vi "8-Axis RS Coordinate Move (bad).vi"() -> ()   [LabVIEW 2013]
uses:
  Typedef/Typedef_Motor_Message.ctl
  EMC API/EMC_Typedef_Motor_Parameters.ctl
  Functional_Global/Typedef_Message_Queue_Action.ctl
  Globals/Global Stop.vi
  <vilib>/Motion/Express/_s/nimc.ex.power.power.axis.vi
  <vilib>/Motion/Express/_s/nimc.ex.resetPosition.resetPosition.axis.vi
  <vilib>/Motion/Express/_s/nimc.ex.straightLineMove.startStraightLineMove.coordinate.modeRelative.0.vi
  Globals/Default Motor Parameters.vi
  <vilib>/Motion/Express/_s/nimc.ex.straightLineMove.startStraightLineMove.axis.modeRelative.0.vi
  <vilib>/Motion/Express/_s/nimc.ex.stopMove.stop.coordinate.modeDecelerate.vi
  <vilib>/Motion/Express/_s/nimc.ex.stopMove.stop.axis.modeDecelerate.vi
  <vilib>/Motion/Express/_s/nimc.ex.read.readTrajectoryData.axis.vi
  <vilib>/Motion/BlockNode/FB.NIMotion.xnode
  Functional_Global/Typedef_FPGA_Interface_Action.ctl
  support/Message Queue/Message Queue.lvlib
  Typedef/Typedef_Coordinate_Move_Message.ctl
panel:
  in  "velocity 3":dbl=1000.0
  in  "position":dbl=1000.0
  in  "velocity 2":dbl=1000.0
  in  "position[]":dbl[](array[numeric])
  in  "Stop all motors 2":bool
  out "error out 2":errorcluster
  in  "velocity":dbl
  in  "# whole revs":dbl=3.0 format="%#_13g"
  in  "Auto Cycle Time (s)":dbl=10.0 format="%#_13g"
  in  "Auto":bool=TRUE
  in  "Mode":enum16{"Seq 1", "Seq 2", "Seq 3"}(ring)
  in  "cts per rev":dbl=1600.0 format="%#_13g"
  in  "Stop all motors":bool
  in  "Max delay (ms)":u32=1000
  in  "Motion Parameters (Min)":T1={"position"=-10000.0, "velocity"=-10000.0, "acceleration"=50000.0, "deceleration"=50000.0, "accel. jerk"=800000.0, "decel. jerk"=800000.0}
  in  "Motion Parameters (Max)":T1={"position"=10000.0, "velocity"=10000.0, "acceleration"=100000.0, "deceleration"=100000.0, "accel. jerk"=1000000.0, "decel. jerk"=1000000.0}
  in  "Command Array":string[](array[string])=["ABS Pos Move", "REL Pos Move", "Velocity Move"]
  out "Command":T2={"Axis"="", "Motion Parameters"={"position"=1000.0, "velocity"=1000.0, "acceleration"=10000.0, "deceleration"=10000.0, "accel. jerk"=10000.0, "decel. jerk"=10000.0}}
  out "Message":string
  out "# elements in queue":i32
  out "error out":errorcluster
  out "Axis Positions":T3(graph)
  out "Axis Velocities":T3(graph)
  out "Array":dbl[](array[knob]) scale=0.0..1600.0
  in  "stop":bool
  # "This example demonstrates how to set up an multi-axis SW architecture using SoftMotion.  You can have state machines that \"produce\" the motion commands, and the consumer will then digest them one at a time.\n\nIn this example, 3 producer loops generate random motion commands at random times (within 1000ms each iteration.) This VI is also meant as a stress test to see if the SM engine is robust enough for complex sequences of motion commands."
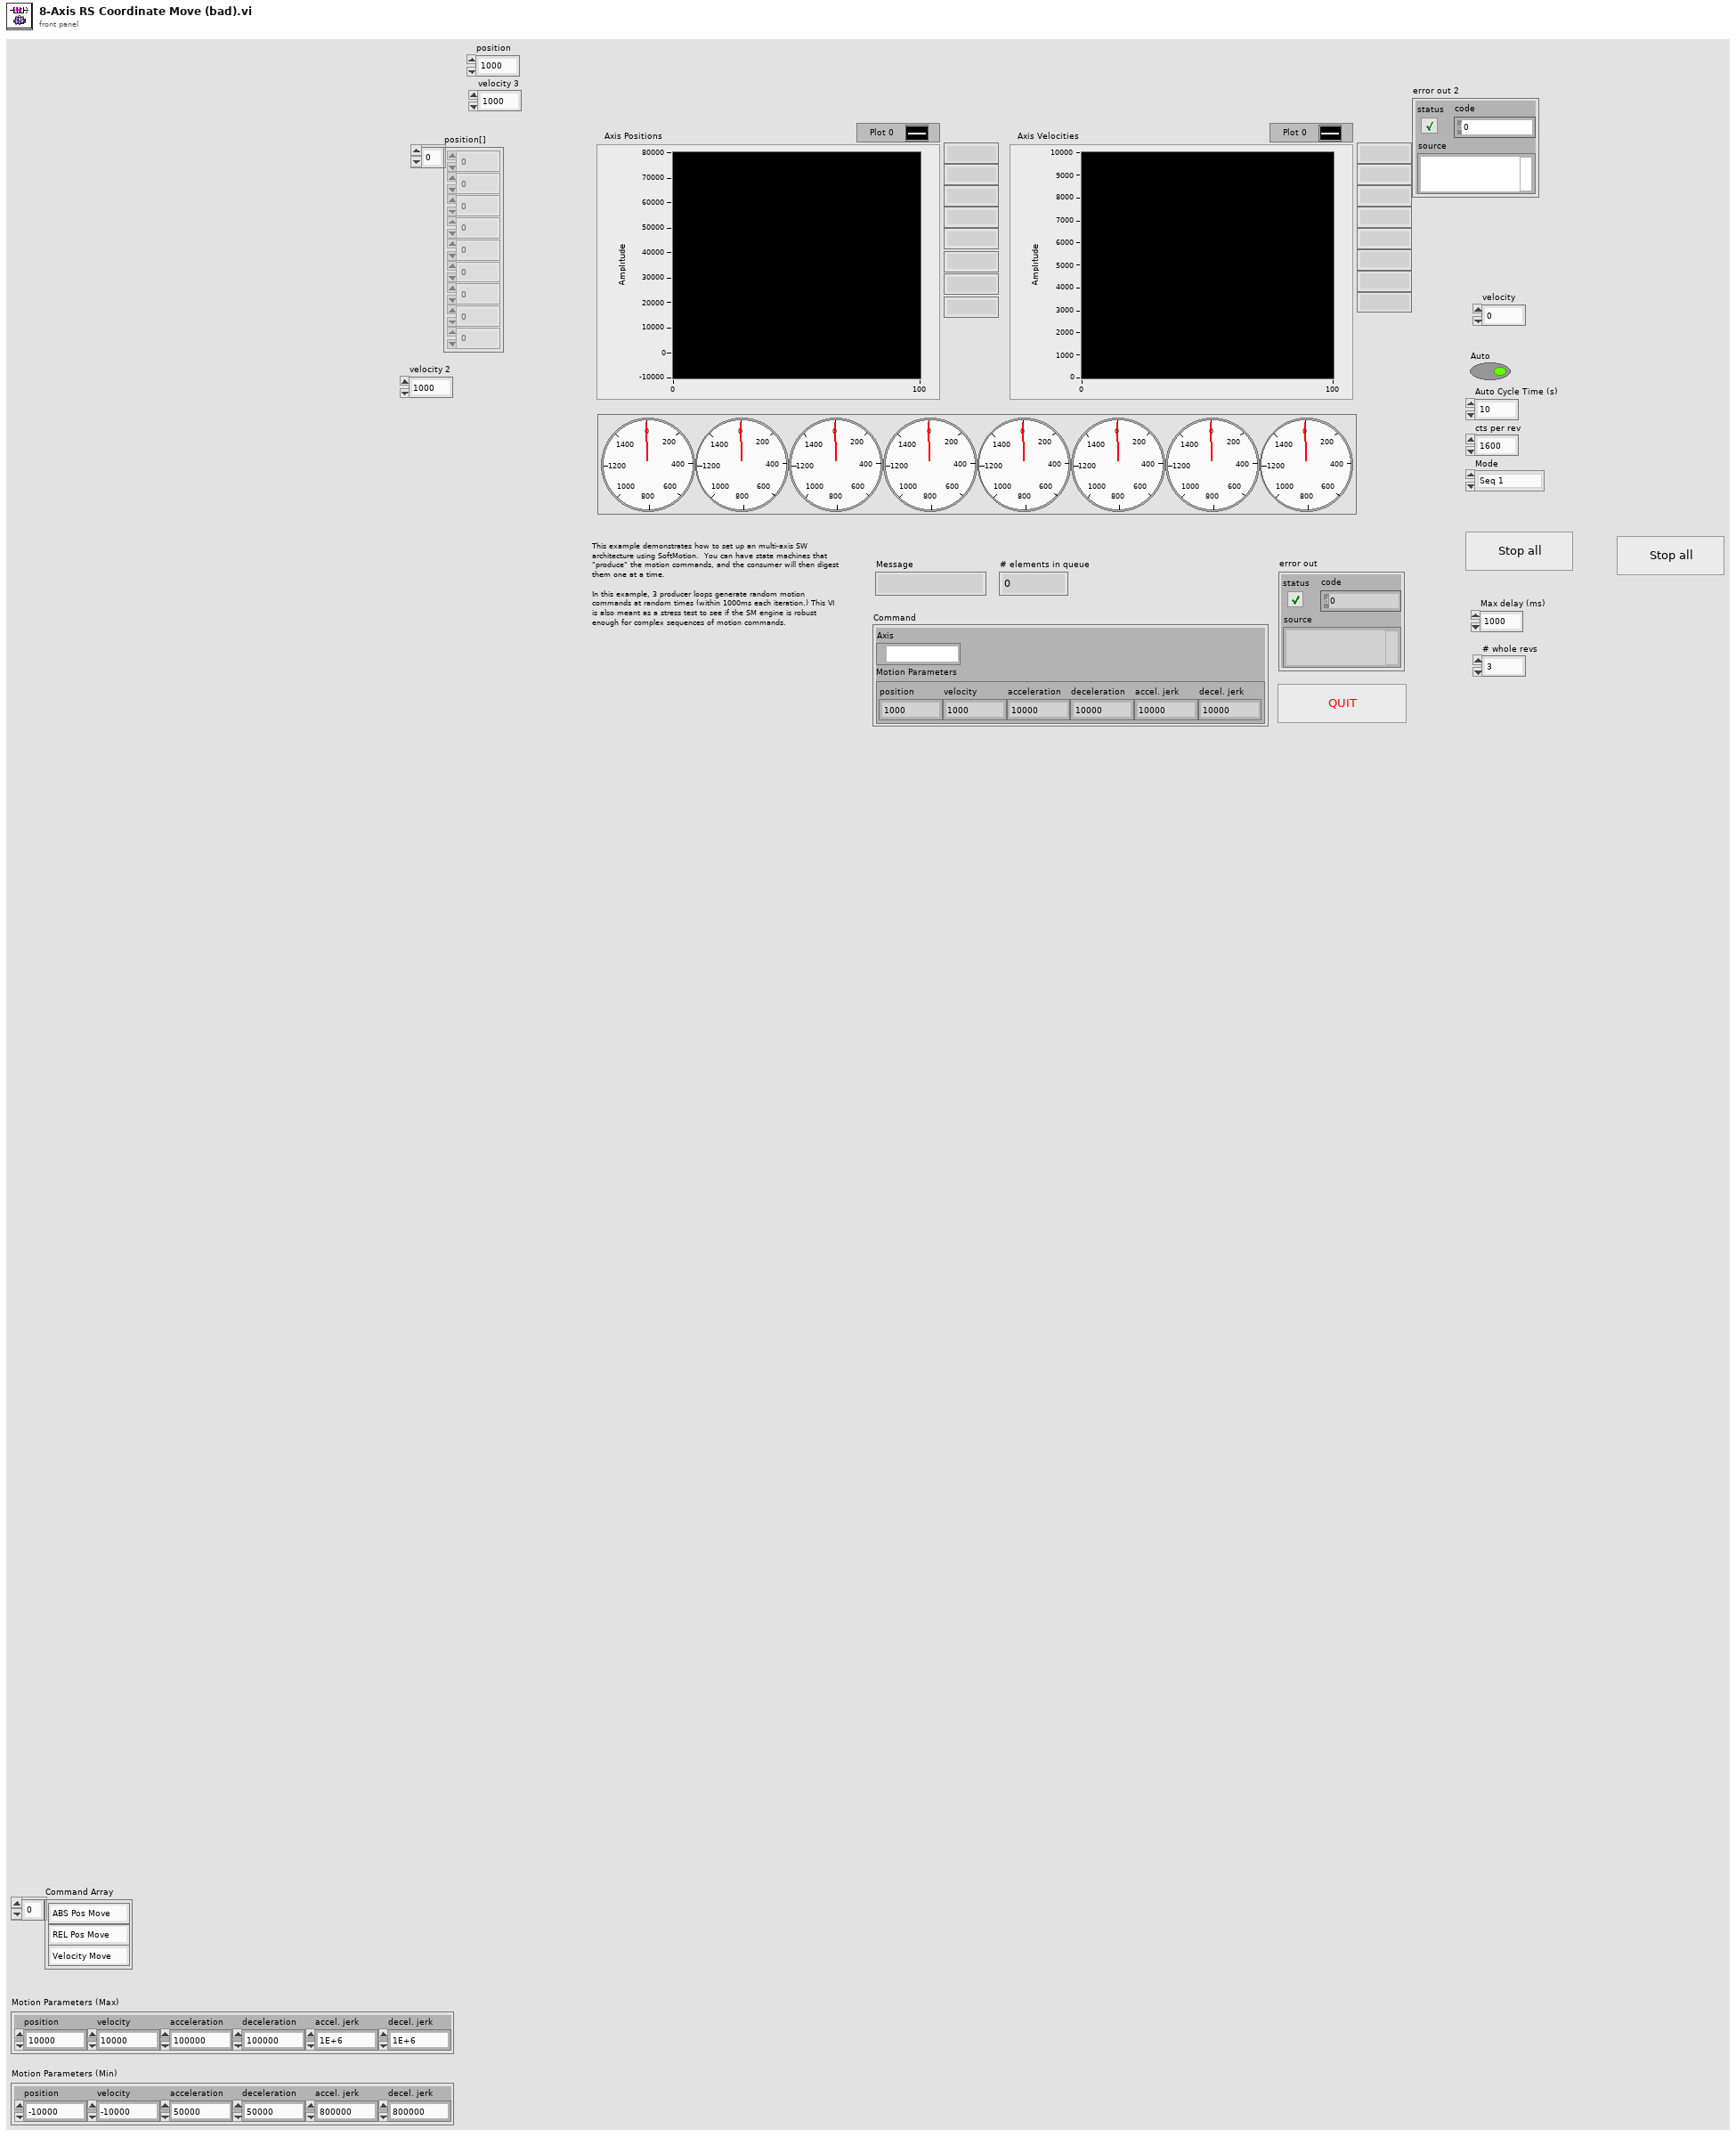
[diagram p1: front panel]
types:
  T1 = typedef "EMC_Typedef_Motor_Parameters.ctl" = cluster{"position":dbl, "velocity":dbl, "acceleration":dbl, "deceleration":dbl, "accel. jerk":dbl, "decel. jerk":dbl}
  T2 = typedef "Typedef_Motor_Message.ctl" = cluster{"Axis":refnum<k21>, "Motion Parameters":T1}
  T3 = cluster{"[0]":dbl, "[1]":dbl, "[2]":dbl, "[3]":dbl, "[4]":dbl, "[5]":dbl, "[6]":dbl, "[7]":dbl}
  T4 = typedef "Typedef_Message_Queue_Action.ctl" = enum16{"Init MQueue", "Get MQueue Ref", "Close MQueue"}
  T5 = typedef "Typedef_FPGA_Interface_Action.ctl" = enum16{"Initialize FPGA", "Get FPGA Reference", "Close FPGA"}
  T6 = typedef "Message Queue.lvlib/Message Cluster.ctl" = cluster{"Message":string, "Message Data":variant}
  T7 = typedef "Typedef_Coordinate_Move_Message.ctl" = cluster{"position[]":dbl[], "velocity":dbl, "Motion Parameters":T1}
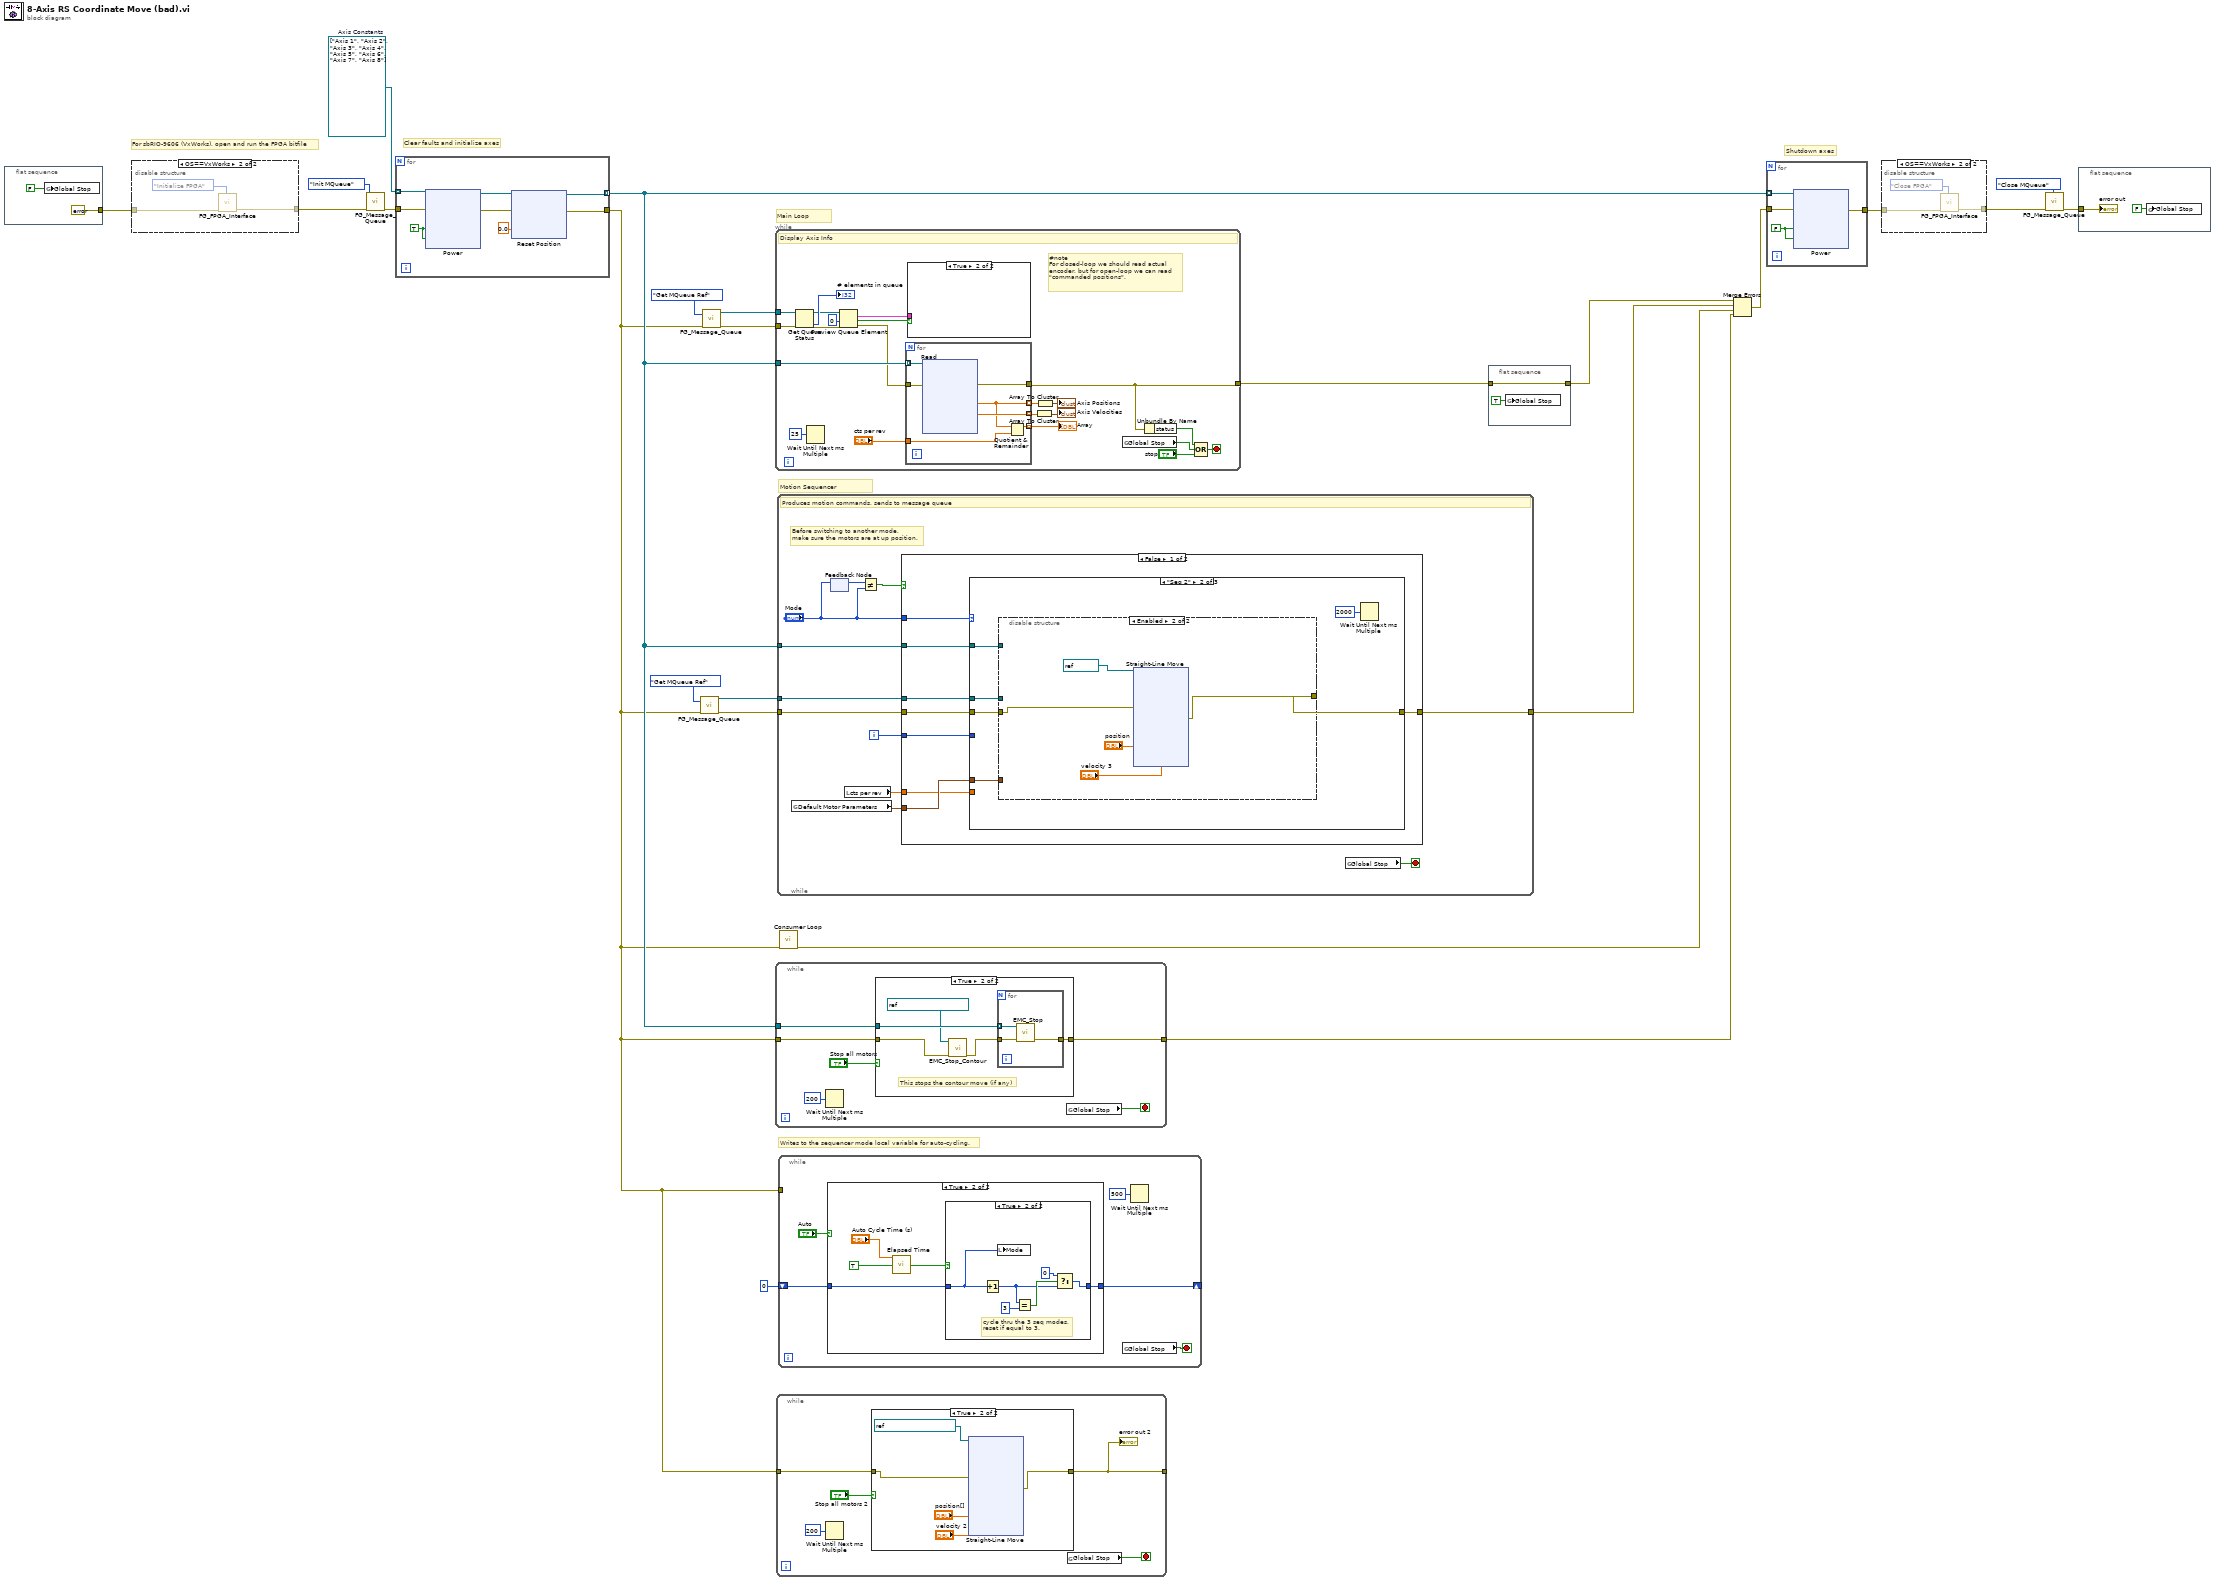
[diagram p0: block diagram]
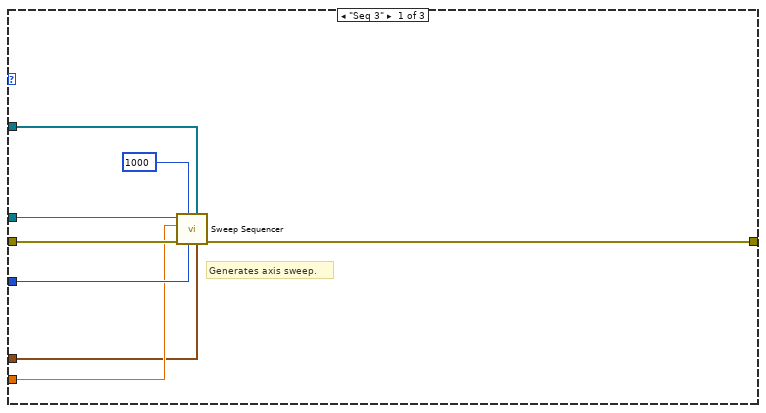
[diagram p2: hidden frame]
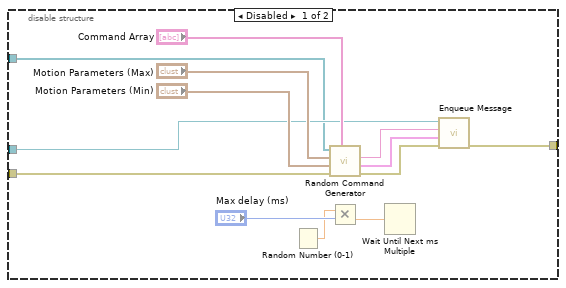
[diagram p3: hidden frame]
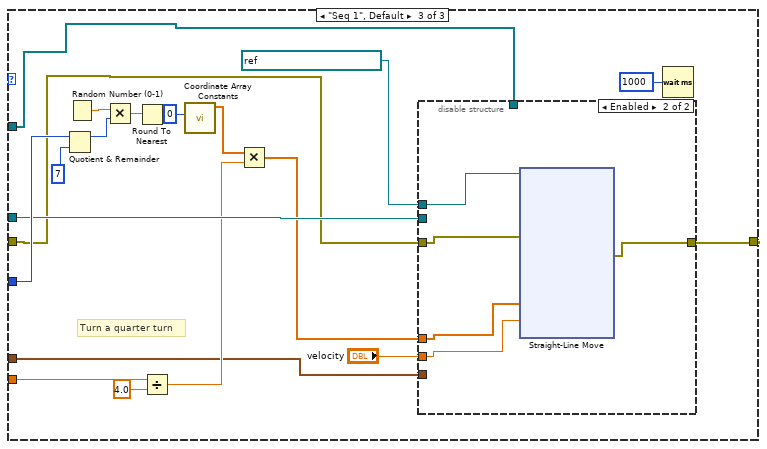
[diagram p4: hidden frame]
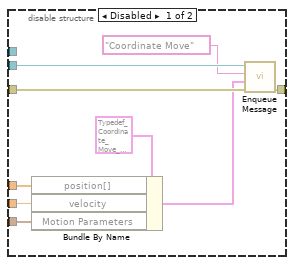
[diagram p5: hidden frame]
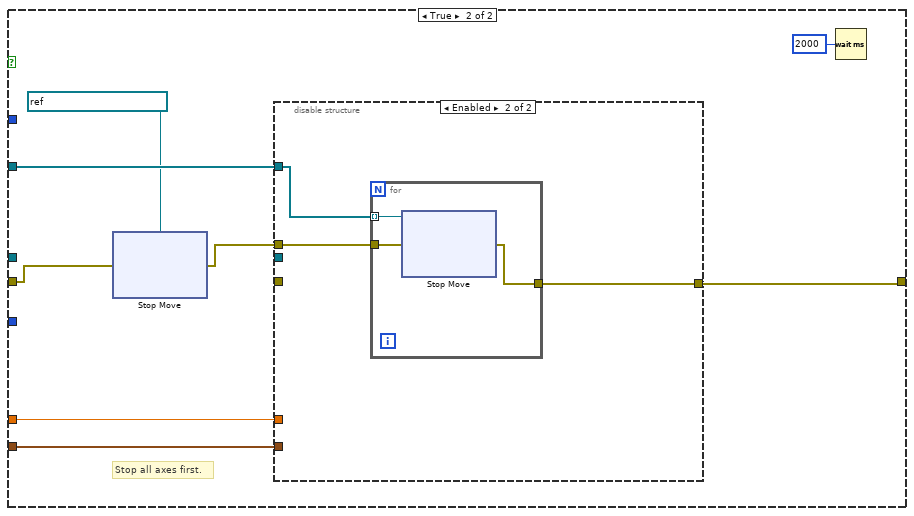
[diagram p6: hidden frame]
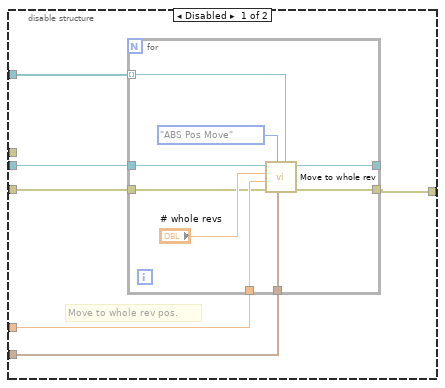
[diagram p7: hidden frame]
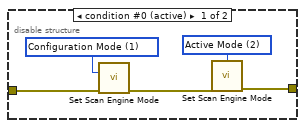
[diagram p13: hidden frame]
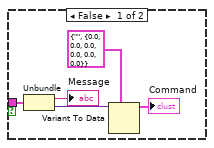
[diagram p14: hidden frame]
diagram:
  w23 = refnum<k21>[] ["Axis 1", "Axis 2", "Axis 3", "Axis 4", "Axis 5", "Axis 6", "Axis 7", "Axis 8"]  # Axis Constants
  # "Motion Sequencer"
  # "Writes to the sequencer mode local variable for auto-cycling."
  # "For sbRIO-9606 (VxWorks), open and run the FPGA bitfile"
  # "Shutdown axes"
  # "Main Loop"
  # "Clear faults and initialize axes"
  n1 = flat-sequence {
    tunnel: [errorcluster {"status"=FALSE, "code"=0, "source"=""} ("error in (no error)")] -> w24
    frame #0 {
      n2 = global write "Global Stop.vi" "Global Stop"(FALSE ("stop")) -> ()
    }
  }
  n3 = disable-structure shown="OS==VxWorks" {
    disable-tunnel: [w31 w32] -> w19
    disable-tunnel: w24 -> [w30 w33]
    frame condition #0 (active) {
      w27 = 1 items=["Configuration Mode"=1, "Active Mode"=2] ("mode (Active Mode)")
      w28 = 2 items=["Configuration Mode"=1, "Active Mode"=2] ("mode (Active Mode)")
      n4 = call <vilib>:"Set Scan Engine Mode.vi"("mode (Active Mode)"=w27, "error in (no error)"=w30) -> ("error out"=w29:errorcluster)  [unwired: 13 in]
      n5 = call <vilib>:"Set Scan Engine Mode.vi"("mode (Active Mode)"=w28, "error in (no error)"=w29) -> ("error out"=w31:errorcluster)  [unwired: 13 in]
    }
    frame condition #1 {
      n6 = call "FG_FPGA_Interface.vi"("Action"=Typedef_FPGA_Interface_Action."Initialize FPGA", "error in"=w33) -> ("error out"=w32:errorcluster)  [unwired: 9 in]
    }
  }
  n7 = call "FG_Message_Queue.vi"("Action"=Typedef_Message_Queue_Action."Init MQueue", "error in"=w19) -> ("error out"=w18:errorcluster)  [unwired: 8 in, 1 out]
  n8 = for {
    tunnel: [w39] -> w1
    tunnel: [w37] -> w4 mode=indexing
    tunnel: w18 -> [w35]
    tunnel: w23 -> [w36] mode=indexing
    w42 = TRUE ("enable axis")
    n9 = xnode ("Power")("enable axis"=w42, "enable drive"=w42, "resource"=w36, "error in"=w35) -> ("resource out"=w38:refnum<k21>, "error out"=w40:errorcluster)
    n10 = xnode ("Reset Position")("position"=0.0, "resource"=w38, "error in"=w40) -> ("resource out"=w37:refnum<k21>, "error out"=w39:errorcluster)
  }
  n11 = call "FG_Message_Queue.vi"("Action"=Typedef_Message_Queue_Action."Get MQueue Ref", "error in"=w1) -> ("error out"=w7:errorcluster, "Message Queue"=w6:refnum<queue>)  [unwired: 8 in]
  n12 = call "FG_Message_Queue.vi"("Action"=Typedef_Message_Queue_Action."Get MQueue Ref", "error in"=w1) -> ("error out"=w10:errorcluster, "Message Queue"=w11:refnum<queue>)  [unwired: 8 in]
  n13 = while {
    tunnel: w10 -> [w66]
    tunnel: w4 -> [w76]
    tunnel: [w60] -> w21
    tunnel: w11 -> [w68]
    stop <- w69 stop-if-true
    # "#note \nFor closed-loop we should read actual \nencoder, but for open-loop we can read\n\"commanded positions\"."
    # "Display Axis Info"
    n14 = Get Queue Status(queue=w68, error in (no error)=w66) -> (queue out=w62:refnum<queue>, error out=w64:errorcluster, # elements in queue=→"# elements in queue":i32)  [unwired: 1 in, 5 out]
    n15 = Wait Until Next ms Multiple(millisecond multiple=u32 25) -> ()  [unwired: 1 out]
    n16 = Preview Queue Element(queue=w62, timeout in ms (-1)=0, error in (no error)=w64) -> (element=w61:T6, timed out?=w59:bool, error out=w63:errorcluster)  [unwired: 1 out]
    n17 = for {
      tunnel: [w91] -> w60
      tunnel: [w87] -> w74 mode=indexing
      tunnel: [w90] -> w79 mode=indexing
      tunnel: w63 -> [w89]
      tunnel: w76 -> [w88] mode=indexing
      tunnel: [w86] -> w75 mode=indexing
      tunnel: "cts per rev" -> [w85]
      n18 = xnode ("Read")("resource"=w88, "error in"=w89) -> ("commanded position"=w87:dbl, "commanded vel."=w90:dbl, "error out"=w91:errorcluster)  [unwired: 2 out]
      n19 = Quotient & Remainder(x=w87, y=w85) -> (x-y*floor(x/y)=w86:dbl)  [unwired: 1 out]
    }
    "Array" <- w75
    n20 = case shown="True" w59 {
      tunnel: w61 -> [w84 _]
      frame False {
        n21 = Unbundle(w84) -> ("Message"=→"Message":string, "Message Data"=w81:variant)
        n22 = Variant To Data(type=T2 {"Axis"="", "Motion Parameters"={"position"=0.0, "velocity"=0.0, "acceleration"=0.0, "deceleration"=0.0, "accel. jerk"=0.0, "decel. jerk"=0.0}} ("Motor_Message"), Variant=w81) -> (data=→"Command":T2)  [unwired: 1 in, 1 out]
      }
      frame True {
      }
    }
    n23 = Array To Cluster(array=w79) -> (cluster=→"Axis Velocities":T3)
    n24 = Array To Cluster(array=w74) -> (cluster=→"Axis Positions":T3)
    n25 = global read "Global Stop.vi" "Global Stop"() -> (w70:bool)
    n26 = Unbundle By Name(w60) -> ("status"=w71:bool)
    n27 = Compound Arithmetic op=OR(w71, w70, "stop") -> (w69:bool)
  }
  n28 = while {
    tunnel: w1 -> [w104]
    tunnel: w4 -> [w102]
    tunnel: [w101] -> w3
    stop <- w100 stop-if-true
    n29 = Wait Until Next ms Multiple(millisecond multiple=u32 200) -> ()  [unwired: 1 out]
    n30 = case shown="True" "Stop all motors" {
      tunnel: w104 -> [w105 w108]
      tunnel: [w105 w110] -> w101
      tunnel: w102 -> [_ w109]
      frame False {
      }
      frame True {
        # "This stops the contour move (if any)"
        n31 = call "EMC_Stop_Contour.vi"("error in (no error)"=w108, "coordinate"=refnum<k21> "Coordinate Space 1") -> ("error out"=w106:errorcluster)  [unwired: 9 in]
        n32 = for {
          tunnel: w106 -> [w113]
          tunnel: w109 -> [w111] mode=indexing
          tunnel: [w112] -> w110
          n33 = call "EMC_Stop.vi"("error in (no error)"=w113, "axis"=w111) -> ("error out"=w112:errorcluster)  [unwired: 8 in, 1 out]
        }
      }
    }
    n34 = global read "Global Stop.vi" "Global Stop"() -> (w100:bool)
  }
  n35 = while {
    tunnel: w1 -> [w118]
    tunnel: [w114] -> _
    stop <- w116 stop-if-true
    n36 = Wait Until Next ms Multiple(millisecond multiple=u32 200) -> ()  [unwired: 1 out]
    n37 = case shown="True" "Stop all motors 2" {
      tunnel: w118 -> [w119 w120]
      tunnel: [w119 w121] -> w114
      frame False {
      }
      frame True {
        n38 = xnode ("Straight-Line Move")("position[]"="position[]", "velocity"="velocity 2", "resource"=refnum<k21> "Coordinate Space 1", "error in"=w120) -> ("error out"=w121:errorcluster)  [unwired: 6 in, 2 out]
      }
    }
    "error out 2" <- w114
    n39 = global read "Global Stop.vi" "Global Stop"() -> (w116:bool)
  }
  n40 = while {
    tunnel: w4 -> [w147]
    tunnel: w7 -> [w149]
    tunnel: w6 -> [w148]
    tunnel: [w145] -> w5
    i -> [w146]
    stop <- w150 stop-if-true
    # "Before switching to another mode,\nmake sure the motors are at up position."
    # "Produces motion commands, sends to message queue"
    n41 = global read "Default Motor Parameters.vi" "Default Motor Parameters"() -> (w142:T1)
    n42 = feedback-in #1("Mode") -> ()
    n43 = feedback #1() -> (w144:enum16{"Seq 1", "Seq 2", "Seq 3"})  [unwired: 1 in]
    n44 = local read "cts per rev"() -> (w140:dbl)
    n45 = Not Equal?(x=w144, y="Mode") -> (x != y?=w143:bool)
    n46 = case shown="False" w143 {
      tunnel: w149 -> [w158 w255]
      tunnel: w148 -> [w157 _]
      tunnel: w147 -> [w156 w258]
      tunnel: w146 -> [w155 _]
      tunnel: [w154 w257] -> w145
      tunnel: "Mode" -> [w153 _]
      tunnel: w142 -> [w152 w260]
      tunnel: w140 -> [w151 w259]
      frame False {
        n47 = case shown="\"Seq 2\"" w153 {
          tunnel: w158 -> [w166 w172 w207]
          tunnel: w157 -> [w164 w171 w221]
          tunnel: w156 -> [w162 w170 w208]
          tunnel: w155 -> [w165 _ w223]
          tunnel: [w163 w169 w222] -> w154
          tunnel: w152 -> [w159 w168 w212]
          tunnel: w151 -> [w160 _ w216]
          frame "Seq 3" {
            # "Generates axis sweep."
            n48 = call "Sweep Sequencer.vi"("Default Motor Parameters"=w159, "Axis Array"=w162, "Loop counter in"=w165, "Max delay (ms)"=u32 1000, "error in (no error)"=w166, "cts per rev"=w160, "Message Queue"=w164) -> ("error out"=w163:errorcluster)  [unwired: 4 in]
          }
          frame "Seq 2" {
            n49 = disable-structure shown="Enabled" {
              disable-tunnel: w172 -> [w179 w187]
              disable-tunnel: w171 -> [w178 _]
              disable-tunnel: w170 -> [w177 _]
              disable-tunnel: [w176 w186] -> w169
              disable-tunnel: w168 -> [_ _]
              frame Disabled {
                n50 = Random Number (0-1)() -> (number: 0 to 1=w174:dbl)
                n51 = call "Random Command Generator.vi"("Command Array"="Command Array", "error in (no error)"=w179, "Motion Parameters (Min)"="Motion Parameters (Min)", "Motion Parameters (Max)"="Motion Parameters (Max)", "Axis Resources"=w177) -> ("error out"=w180:errorcluster, "Motor_Message"=w182:T2, "Command Out"=w181:string)  [unwired: 4 in]
                n52 = Multiply(x=w174, y="Max delay (ms)") -> (x*y=w173:dbl)
                n53 = Wait Until Next ms Multiple(millisecond multiple=w173) -> ()  [unwired: 1 out]
                n54 = call "Enqueue Message.vi"("error in (no error)"=w180, "Message Data"=w182, "Message"=w181, "Message Queue"=w178) -> ("error out"=w176:errorcluster)  [unwired: 6 in, 1 out]
              }
              frame Enabled {
                n55 = xnode ("Straight-Line Move")("position"="position", "velocity"="velocity 3", "resource"=refnum<k21> "Axis 1", "error in"=w187) -> ("error out"=w186:errorcluster)  [unwired: 6 in, 2 out]
              }
            }
            n56 = Wait Until Next ms Multiple(millisecond multiple=u32 2000) -> ()  [unwired: 1 out]
          }
          frame "Seq 1", Default {
            # "Turn a quarter turn"
            n57 = Quotient & Remainder(x=w223, y=7) -> (x-y*floor(x/y)=w218:i32)  [unwired: 1 out]
            n58 = Random Number (0-1)() -> (number: 0 to 1=w219:dbl)
            n59 = Multiply(x=w219, y=w218) -> (x*y=w217:dbl)
            n60 = Round To Nearest(number=w217) -> ()  [unwired: 1 out]
            n61 = Divide(x=w216, y=4.0) -> (x/y=w213:dbl)
            n62 = call "Coordinate Array Constants.vi"("Numeric"=0) -> ("Axis Positions"=w214:dbl[])  [unwired: 10 in]
            n63 = Multiply(x=w214, y=w213) -> (x*y=w211:dbl[])
            n64 = disable-structure shown="Enabled" {
              disable-tunnel: w207 -> [w233 w235]
              disable-tunnel: [w232 w234] -> w222
              disable-tunnel: w221 -> [w231 _]
              disable-tunnel: w212 -> [w227 _]
              disable-tunnel: w211 -> [w226 w237]
              disable-tunnel: "velocity" -> [w225 w236]
              disable-tunnel: refnum<k21> "Coordinate Space 1" ("resource") -> [_ w238]
              disable-tunnel: w208 -> [_ _]
              frame Disabled {
                n65 = Bundle By Name(cluster=T7 {"position[]"=[], "velocity"=1000.0, "Motion Parameters"={"position"=1000.0, "velocity"=1000.0, "acceleration"=10000.0, "deceleration"=10000.0, "accel. jerk"=10000.0, "decel. jerk"=10000.0}} ("Coordinate_Move_Message"), "position[]"=w226, "velocity"=w225, "Motion Parameters"=w227) -> (w230:T7)
                n66 = call "Enqueue Message.vi"("error in (no error)"=w233, "Message Data"=w230, "Message"="Coordinate Move", "Message Queue"=w231) -> ("error out"=w232:errorcluster)  [unwired: 6 in, 1 out]
              }
              frame Enabled {
                n67 = xnode ("Straight-Line Move")("position[]"=w237, "velocity"=w236, "resource"=w238, "error in"=w235) -> ("error out"=w234:errorcluster)  [unwired: 6 in, 2 out]
              }
            }
            n68 = Wait (ms)(milliseconds to wait=u32 1000) -> ()  [unwired: 1 out]
          }
        }
      }
      frame True {
        # "Stop all axes first."
        n69 = xnode ("Stop Move")("resource"=refnum<k21> "Coordinate Space 1", "error in"=w255) -> ("error out"=w254:errorcluster)  [unwired: 1 in, 2 out]
        n70 = disable-structure shown="Enabled" {
          disable-tunnel: w260 -> [w275 _]
          disable-tunnel: w259 -> [w274 _]
          disable-tunnel: w258 -> [w273 w286]
          disable-tunnel: _ -> [w272 _]
          disable-tunnel: _ -> [w271 _]
          disable-tunnel: [w270 w285] -> w257
          disable-tunnel: w254 -> [_ w287]
          frame Disabled {
            # "Move to whole rev pos."
            n71 = for {
              tunnel: w273 -> [w282] mode=indexing
              tunnel: [w284] -> w270
              tunnel: w275 -> [w281]
              tunnel: w274 -> [w280]
              tunnel: [w278] -> _
              tunnel: w272 -> [w277]
              tunnel: w271 -> [w276]
              n72 = call "Move to whole rev.vi"("resource in"=w282, "Default Motor Parameters"=w281, "Mode"=enum16{"ABS Pos Move", "REL Pos Move"}."ABS Pos Move", "error in (no error)"=w276, "cts per rev"=w280, "# whole revs"="# whole revs", "Queue in"=w277) -> ("error out"=w284:errorcluster, "Queue out"=w278:refnum<queue>)  [unwired: 3 in]
            }
          }
          frame Enabled {
            n73 = for {
              tunnel: w287 -> [w290]
              tunnel: w286 -> [w289] mode=indexing
              tunnel: [w288] -> w285
              n74 = xnode ("Stop Move")("resource"=w289, "error in"=w290) -> ("error out"=w288:errorcluster)  [unwired: 1 in, 2 out]
            }
          }
        }
        n75 = Wait (ms)(milliseconds to wait=u32 2000) -> ()  [unwired: 1 out]
      }
    }
    n76 = global read "Global Stop.vi" "Global Stop"() -> (w150:bool)
  }
  n77 = while {
    tunnel: w1 -> [_]
    shift-right: [w300] -> _
    shift-left: 0 -> [w301]
    stop <- w303 stop-if-true
    n78 = case shown="True" "Auto" {
      tunnel: w301 -> [w304 w307]
      tunnel: [w304 w306] -> w300
      frame False {
      }
      frame True {
        n79 = call "Elapsed Time"("Time Target (s)"="Auto Cycle Time (s)", "Auto Reset"=TRUE) -> ("Time has Elapsed"=w308:bool)  [unwired: 10 in, 7 out]
        n80 = case shown="True" w308 {
          tunnel: w307 -> [w310 w316]
          tunnel: [w310 w311] -> w306
          frame False {
          }
          frame True {
            # "cycle thru the 3 seq modes,\nreset if equal to 3."
            n81 = Increment(x=w316) -> (x+1=w313:i32)
            n82 = local write "Mode"(w316) -> ()
            n83 = Equal?(x=w313, y=3) -> (x = y?=w314:bool)
            n84 = Select(t=0, s=w314, f=w313) -> (s? t:f=w311:i32)
          }
        }
      }
    }
    n85 = global read "Global Stop.vi" "Global Stop"() -> (w303:bool)
    n86 = Wait Until Next ms Multiple(millisecond multiple=u32 500) -> ()  [unwired: 1 out]
  }
  n87 = call "Consumer Loop.vi"("error in (no error)"=w1) -> ("error out"=w9:errorcluster)  [unwired: 10 in]
  n88 = flat-sequence {
    tunnel: w21 -> [w317]
    tunnel: [w317] -> w13
    frame #0 {
      n89 = global write "Global Stop.vi" "Global Stop"(TRUE ("stop")) -> ()
    }
  }
  n90 = Merge Errors(w13, w5, w9, w3) -> (w17:errorcluster)
  n91 = for {
    tunnel: w4 -> [w322] mode=indexing
    tunnel: [w320] -> w22
    tunnel: w17 -> [w319]
    w321 = FALSE ("enable axis")
    n92 = xnode ("Power")("enable axis"=w321, "enable drive"=w321, "resource"=w322, "error in"=w319) -> ("error out"=w320:errorcluster)  [unwired: 1 out]
  }
  n93 = disable-structure shown="OS==VxWorks" {
    disable-tunnel: [w333 w334] -> w15
    disable-tunnel: w22 -> [w333 w335]
    frame condition #0 (active) {
    }
    frame condition #1 {
      n94 = call "FG_FPGA_Interface.vi"("Action"=Typedef_FPGA_Interface_Action."Close FPGA", "error in"=w335) -> ("error out"=w334:errorcluster)  [unwired: 9 in]
    }
  }
  n95 = call "FG_Message_Queue.vi"("Action"=Typedef_Message_Queue_Action."Close MQueue", "error in"=w15) -> ("error out"=w14:errorcluster)  [unwired: 8 in, 1 out]
  n96 = flat-sequence {
    tunnel: w14 -> [w337]
    frame #0 {
      n97 = global write "Global Stop.vi" "Global Stop"(FALSE ("stop")) -> ()
      "error out" <- w337
    }
  }
